vi "ADC温度采集实验.vi"() -> ()   [LabVIEW 2011]
uses:
  <vilib>/STM32_DriverVI_Interface_F4/ADC/ADC123_Period_Interface_F4.ctl
  <vilib>/eio/EIO_TerminalDirection.ctl
  <vilib>/STM32_DriverVI_Interface/ADC/ADC1_Channel_Interface.ctl
  <vilib>/STM32_DriverVI_Interface_F4/ADC_EIO/ADC1_EIO_Interface_F4.vi
  <vilib>/STM32_DriverVI_Interface_F4/GPIO_EIO/GPO_EIO_Inner_F4.vi
  <vilib>/eio/EIONode/EIONode.xnode
panel:
  in  "输入变量":dbl
  out "STM32_TEMP_V":sgl
  out "输出变量":dbl
  in  "停止":bool
  out "数值":i32
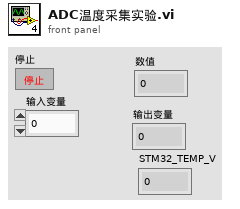
[diagram p1: front panel]
types:
  T1 = enum8{"P0", "P1", "P2", "P3", "P4", "P5", "P6", "P7", "P8", "P9", "P10", "P11", "P12", "P13", "P14", "P15"}
  T2 = typedef "ADC123_Period_Interface_F4.ctl" = enum8{"0.71 us", "1.28 us", "1.90 us", "3.24 us", "4.57 us", "5.90 us", "7.43 us", "23.4 us"}
  T3 = typedef "ADC1_Channel_Interface.ctl" = enum8{"Channel_0（PA0）", "Channel_1（PA1）", "Channel_2（PA2）", "Channel_3（PA3）", "Channel_4（PA4）", "Channel_5（PA5）", "Channel_6（PA6）", "Channel_7（PA7）", "Channel_8（PB0）", "Channel_9（PB1）", "Channel_10（PC0）", "Channel_11（PC1）", "Channel_12（PC2）", "Channel_13（PC3）", "Channel_14（PC4）", "Channel_15（PC5）", "Channel_16（Temperature_Inner）", "Channel_17（Voltage_Ref_Inner）"}
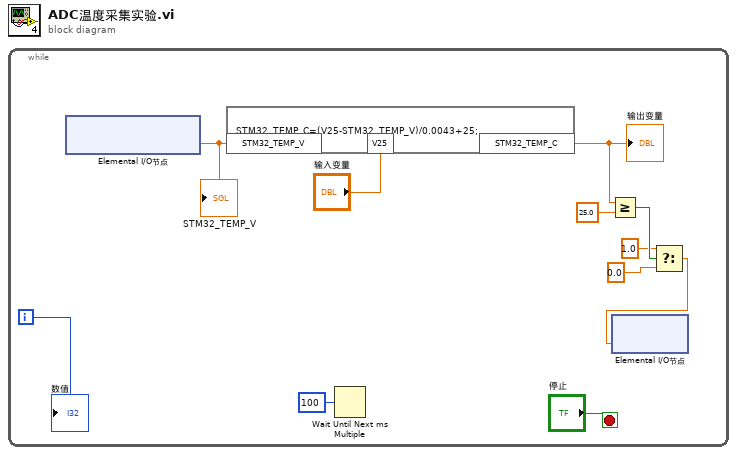
[diagram p0: block diagram]
diagram:
  n1 = while {
    i -> [w10]
    stop <- "停止" stop-if-true
    n2 = xnode "Elemental I/O节点"() -> ("STM32_TEMP_V"=w11:sgl)  [unwired: 1 in, 1 out]
    "STM32_TEMP_V" <- w11
    n3 = formula code="STM32_TEMP_C=(V25-STM32_TEMP_V)/0.0043+25;"("STM32_TEMP_V"=w11, "V25"="输入变量") -> ("STM32_TEMP_C"=w7:dbl)
    "输出变量" <- w7
    n4 = Wait Until Next ms Multiple(millisecond multiple=u32 100 ("毫秒倍数")) -> ()  [unwired: 1 out]
    n5 = Greater Or Equal?(x=w7, y=25.0) -> (x >= y?=w5:bool)
    n6 = Select(t=1.0, s=w5, f=0.0) -> (s? t:f=w4:dbl)
    n7 = xnode "Elemental I/O节点"("BEEP"=w4) -> ()  [unwired: 1 in, 1 out]
    "数值" <- w10
  }
